vi "CRYMake Calibration Step Default.vi"(8 "Write?":bool, 11 "Hardware flattened":string) -> (3 "Calibration flattened":string)   [LabVIEW 2013]
uses:
  Typedef Control/CRYCalibration 2DCluster.ctl
  Typedef Control/CRYCalibration Cluster.ctl
  Typedef Control/CRYData Cluster.ctl
  Typedef Control/CRYCalibration All Cluster.ctl
  CRYMainGlobal.vi
panel:
  out "OK?":bool
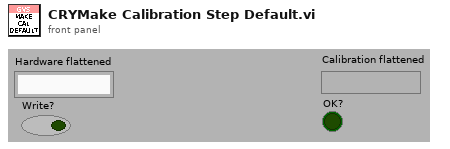
[diagram p1: front panel]
types:
  T1 = typedef "CRYCalibration All Cluster.ctl" = cluster{"Calibration 2D":T2[], "Help":string, "Tab Value":i32, "Input Signal Type":string, "Output Signal Type":string}
  T2 = typedef "CRYCalibration 2DCluster.ctl" = cluster{"Calibration":T3, "Corr Curve":T4, "EQ Curve":T4, "Sens Curve":T4}
  T3 = typedef "CRYCalibration Cluster.ctl" = cluster{"Calibration Step Name":string, "Device":string, "Correction Curve Name":string, "Equalization Curve Name":string, "Sensitivity Curve Name":string, "Corr Folder and File":string, "EQ Folder and File":string, "Sens Folder and File":string, "Corr Step size":u16, "EQ Step size":u16, "Input":bool, "Last Cal Date (sec)":timestamp, "Cha Name":string, "Corr Curve Found":bool, "EQ Curve Found":bool, "Sens Curve Found":bool, "Signal Type":string, "Calibrated Device":string, "Hz":u32}
  T4 = typedef "CRYData Cluster.ctl" = cluster{"Name":string, "Curve":cluster{"x":dbl, "y":dbl, "z":dbl}[], "X data":u16, "Y data":u16, "Z data":u16, "X axis":u16, "Y axis":u16, "Z axis":u16, "X unit":string, "Y unit":string, "Z unit":string, "X dB ref":dbl, "Y dB ref":dbl, "Z dB ref":dbl, "single val":bool, "protected":bool, "display X":bool, "display Y":bool, "display Z":bool, "Test Info":string, "Step No.":i32, "Plot Settings":cluster{"Color":u32, "Interpolation":u8, "Point Style":u8, "Line Style":u8, "Point Color":u32, "Line Width":u8, "Bar Plot Style":u8, "Fill To":i16}, "AutoProtect":bool}
  T5 = cluster{"StepName":string, "setup flattened":string}[]
  T6 = cluster{"StepName":string, "setup flattened":string}
  T7 = enum16{"open", "replace", "create", "open or create", "replace or create", "replace or create with confirmation"}
  T8 = enum16{"big-endian, network order", "native, host order", "little-endian"}
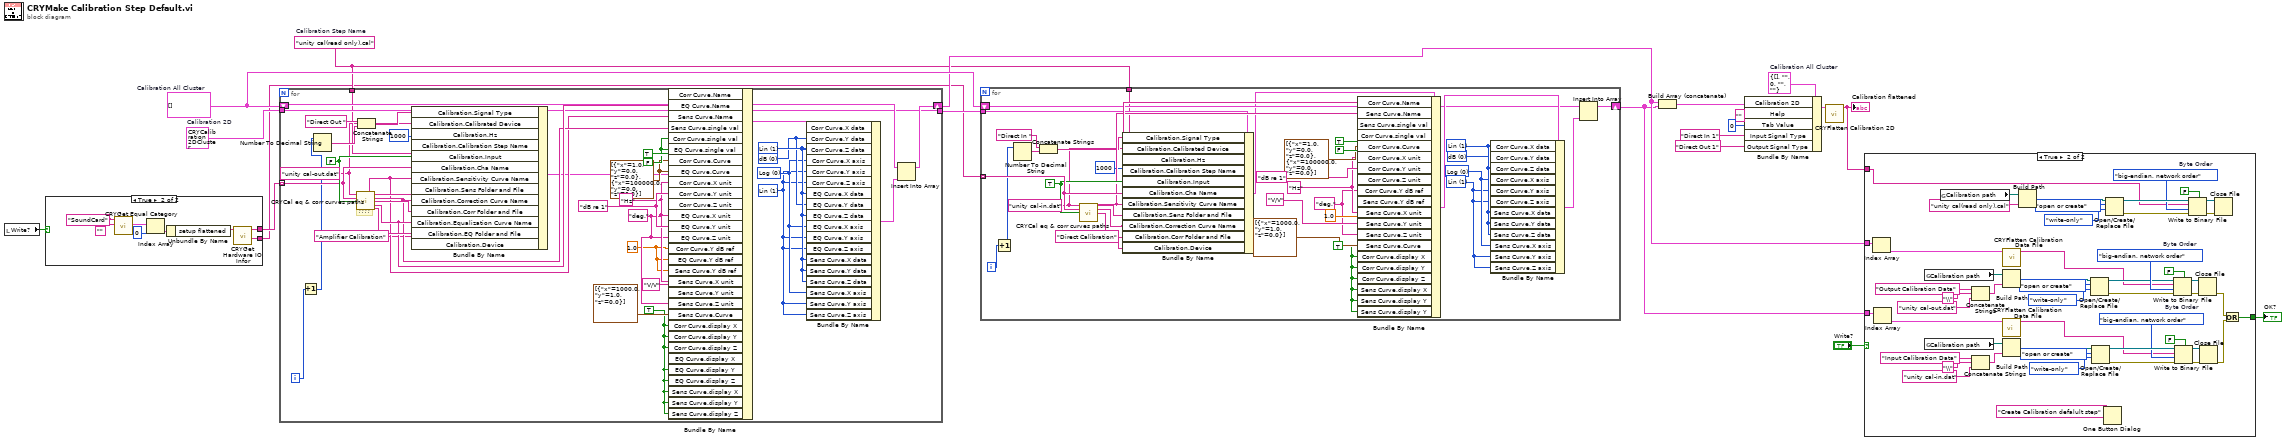
[diagram p0: block diagram]
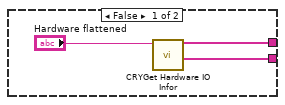
[diagram p2: hidden frame]
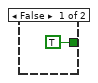
[diagram p3: hidden frame]
diagram:
  w5 = "unity cal(read only).cal"  # Calibration Step Name
  w17 = T1 {"Calibration 2D"=[], "Help"="", "Tab Value"=0, "Input Signal Type"="", "Output Signal Type"=""}  # Calibration All Cluster
  w18 = T2 {"Calibration"={"Calibration Step Name"="", "Device"="", "Correction Curve Name"="", "Equalization Curve Name"="", "Sensitivity Curve Name"="", "Corr Folder and File"="", "EQ Folder and File"="", "Sens Folder and File"="", "Corr Step size"=0, "EQ Step size"=0, "Input"=FALSE, "Last Cal Date (sec)"=timestamp(0 s since 1904-01-01), "Cha Name"="", "Corr Curve Found"=FALSE, "EQ Curve Found"=FALSE, "Sens Curve Found"=FALSE, "Signal Type"="", "Calibrated Device"="", "Hz"=0}, "Corr Curve"={"Name"="", "Curve"=[], "X data"=1, "Y data"=1, "Z data"=1, "X axis"=0, "Y axis"=1, "Z axis"=1, "X unit"="", "Y unit"="", "Z unit"="deg.", "X dB ref"=1.0, "Y dB ref"=1.0, "Z dB ref"=1.0, "single val"=FALSE, "protected"=FALSE, "display X"=FALSE, "display Y"=TRUE, "display Z"=TRUE, "Test Info"="", "Step No."=0, "Plot Settings"={"Color"=0, "Interpolation"=0, "Point Style"=0, "Line Style"=0, "Point Color"=0, "Line Width"=0, "Bar Plot Style"=0, "Fill To"=0}, "AutoProtect"=FALSE}, "EQ Curve"={"Name"="", "Curve"=[], "X data"=1, "Y data"=1, "Z data"=1, "X axis"=0, "Y axis"=1, "Z axis"=1, "X unit"="Hz", "Y unit"="", "Z unit"="deg.", "X dB ref"=1.0, "Y dB ref"=1.0, "Z dB ref"=1.0, "single val"=FALSE, "protected"=FALSE, "display X"=TRUE, "display Y"=TRUE, "display Z"=TRUE, "Test Info"="", "Step No."=0, "Plot Settings"={"Color"=0, "Interpolation"=0, "Point Style"=0, "Line Style"=0, "Point Color"=0, "Line Width"=0, "Bar Plot Style"=0, "Fill To"=0}, "AutoProtect"=FALSE}, "Sens Curve"={"Name"="", "Curve"=[], "X data"=1, "Y data"=1, "Z data"=1, "X axis"=0, "Y axis"=1, "Z axis"=1, "X unit"="Hz", "Y unit"="", "Z unit"="deg.", "X dB ref"=1.0, "Y dB ref"=1.0, "Z dB ref"=1.0, "single val"=FALSE, "protected"=FALSE, "display X"=TRUE, "display Y"=TRUE, "display Z"=TRUE, "Test Info"="", "Step No."=0, "Plot Settings"={"Color"=0, "Interpolation"=0, "Point Style"=0, "Line Style"=0, "Point Color"=0, "Line Width"=0, "Bar Plot Style"=0, "Fill To"=0}, "AutoProtect"=FALSE}}  # Calibration 2D
  w9 = T2[] []  # Calibration All Cluster
  n1 = local read "Write?"() -> (w3:bool)
  n2 = case shown="True" w3 {
    tunnel: [w21 w25] -> w2
    tunnel: [w20 w24] -> w1
    frame False {
      n3 = call "CRYGet Hardware IO Infor.vi"("Hardware setup In"="Hardware flattened") -> ("I_Hardware Channel Name Out"=w20:string[], "O_Hardware Channel Name Out"=w21:string[])  [unwired: 9 out]
    }
    frame True {
      (unwired) ""
      w23 = "SoundCard" ("CategoryName")
      n4 = call "CRYGet Equal Category.vi"("Current StepName"=w23, "Find CategoryName"=w23) -> ("setup flattened Array out"=w27:T5)  [unwired: 9 out]
      n5 = Index Array(array=w27, index=0) -> (element=w28:T6)
      n6 = Unbundle By Name(w28) -> ("setup flattened"=w29:string)
      n7 = call "CRYGet Hardware IO Infor.vi"("Hardware setup In"=w29) -> ("I_Hardware Channel Name Out"=w24:string[], "O_Hardware Channel Name Out"=w25:string[])  [unwired: 9 out]
    }
  }
  n8 = for {
    tunnel: w2 -> [w35] mode=indexing
    shift-right: [w40] -> w7
    shift-left: w9 -> [w41]
    tunnel: w18 -> [w39]
    tunnel: [w39] -> w19
    tunnel: w5 -> [w31]
    i -> [w34]
    w30 = "unity cal-out.dat" ("Step Name")
    w46 = u16 1 items=["Log", "Lin"] ("Y axis")
    w47 = u16 0 items=["Log", "Lin"] ("Y axis")
    w48 = u16 0 items=["dB", "Lin"] ("Y data")
    w49 = u16 1 items=["dB", "Lin"] ("Y data")
    w50 = TRUE ("Corr Curve.display X")
    w56 = 1.0 ("EQ Curve.Y dB ref")
    w57 = "deg." ("Corr Curve.Z unit")
    w60 = "dB re 1" ("Corr Curve.Y unit")
    w59 = "Hz" ("Corr Curve.X unit")
    w61 = cluster{"x":dbl, "y":dbl, "z":dbl}[] [{"x"=1.0, "y"=0.0, "z"=0.0}, {"x"=100000.0, "y"=0.0, "z"=0.0}] ("Corr Curve.Curve")
    w62 = FALSE ("Corr Curve.single val")
    w66 = FALSE ("Input")
    # "????"
    n9 = Increment(x=w34) -> (x+1=w32:i32)
    n10 = Number To Decimal String(number=w32) -> (decimal integer string=w33:string)  [unwired: 1 in]
    n11 = call "CRYCal eq & corr curves paths.vi"("Calibrated Device Name"=w30, "Channel Name"=w35, "In_Out"=w66) -> ("Sens Currve Name"=w51:string, "Sens Curve File"=w65:string, "Corr Curve Name"=w52:string, "Corr Curve File"=w54:string, "EQ Curve Name"=w53:string, "EQ Curve File"=w64:string)  [unwired: 7 out]
    n12 = Concatenate Strings("Direct Out " ("Calibration.Signal Type"), w33) -> (w36:string)
    n13 = Bundle By Name(cluster=w39, "Calibration.Signal Type"=w36, "Calibration.Calibrated Device"=w30, "Calibration.Hz"=u32 1000, "Calibration.Calibration Step Name"=w31, "Calibration.Input"=w66, "Calibration.Cha Name"=w35, "Calibration.Sensitivity Curve Name"=w51, "Calibration.Sens Folder and File"=w65, "Calibration.Correction Curve Name"=w52, "Calibration.Corr Folder and File"=w54, "Calibration.Equalization Curve Name"=w53, "Calibration.EQ Folder and File"=w64, "Calibration.Device"="Amplifier Calibration" ("Device")) -> (w44:T2)
    n14 = Bundle By Name(cluster=w44, "Corr Curve.Name"=w52, "EQ Curve.Name"=w53, "Sens Curve.Name"=w51, "Sens Curve.single val"=TRUE, "Corr Curve.single val"=w62, "EQ Curve.single val"=w62, "Corr Curve.Curve"=w61, "EQ Curve.Curve"=w61, "Corr Curve.X unit"=w59, "Corr Curve.Y unit"=w60, "Corr Curve.Z unit"=w57, "EQ Curve.X unit"=w59, "EQ Curve.Y unit"=w60, "EQ Curve.Z unit"=w57, "Corr Curve.Y dB ref"=w56, "EQ Curve.Y dB ref"=w56, "Sens Curve.Y dB ref"=w56, "Sens Curve.X unit"=w59, "Sens Curve.Y unit"="V/V", "Sens Curve.Z unit"=w57, "Sens Curve.Curve"=cluster{"x":dbl, "y":dbl, "z":dbl}[] [{"x"=1000.0, "y"=1.0, "z"=0.0}], "Corr Curve.display X"=w50, "Corr Curve.display Y"=w50, "Corr Curve.display Z"=w50, "EQ Curve.display X"=w50, "EQ Curve.display Y"=w50, "EQ Curve.display Z"=w50, "Sens Curve.display X"=w50, "Sens Curve.display Y"=w50, "Sens Curve.display Z"=w50) -> (w43:T2)
    n15 = Bundle By Name(cluster=w43, "Corr Curve.X data"=w49, "Corr Curve.Y data"=w48, "Corr Curve.Z data"=w49, "Corr Curve.X axis"=w47, "Corr Curve.Y axis"=w46, "Corr Curve.Z axis"=w46, "EQ Curve.X data"=w49, "EQ Curve.Y data"=w48, "EQ Curve.Z data"=w49, "EQ Curve.X axis"=w47, "EQ Curve.Y axis"=w46, "EQ Curve.Z axis"=w46, "Sens Curve.X data"=w49, "Sens Curve.Y data"=w49, "Sens Curve.Z data"=w49, "Sens Curve.X axis"=w47, "Sens Curve.Y axis"=w46, "Sens Curve.Z axis"=w46) -> (w42:T2)
    n16 = Insert Into Array(array=w41, new element=w42) -> (w40:T2[])  [unwired: 1 in]
  }
  n17 = for {
    tunnel: w1 -> [w101] mode=indexing
    tunnel: w19 -> [w79]
    shift-right: [w77] -> w6
    shift-left: w9 -> [w78]
    tunnel: w5 -> [w69]
    i -> [w75]
    w68 = "unity cal-in.dat" ("Step Name")
    w81 = u16 1 items=["Log", "Lin"] ("Y axis")
    w82 = u16 0 items=["Log", "Lin"] ("Y axis")
    w83 = u16 0 items=["dB", "Lin"] ("Y data")
    w84 = u16 1 items=["dB", "Lin"] ("Y data")
    w86 = TRUE ("Corr Curve.display X")
    w93 = 1.0 ("EQ Curve.Y dB ref")
    w90 = "deg." ("Corr Curve.Z unit")
    w92 = "Hz" ("Corr Curve.X unit")
    w100 = TRUE ("Input")
    n18 = Increment(x=w75) -> (x+1=w70:i32)
    n19 = Number To Decimal String(number=w70) -> (decimal integer string=w74:string)  [unwired: 1 in]
    n20 = Concatenate Strings("Direct In " ("string"), w74) -> (w71:string)
    n21 = call "CRYCal eq & corr curves paths.vi"("Calibrated Device Name"=w68, "Channel Name"=w101, "In_Out"=w100) -> ("Sens Currve Name"=w87:string, "Sens Curve File"=w99:string, "Corr Curve Name"=w88:string, "Corr Curve File"=w98:string)  [unwired: 9 out]
    n22 = Bundle By Name(cluster=w79, "Calibration.Signal Type"=w71, "Calibration.Calibrated Device"=w68, "Calibration.Hz"=u32 1000, "Calibration.Calibration Step Name"=w69, "Calibration.Input"=w100, "Calibration.Cha Name"=w101, "Calibration.Sensitivity Curve Name"=w87, "Calibration.Sens Folder and File"=w99, "Calibration.Correction Curve Name"=w88, "Calibration.Corr Folder and File"=w98, "Calibration.Device"="Direct Calibration" ("Device")) -> (w67:T2)
    n23 = Bundle By Name(cluster=w67, "Corr Curve.Name"=w88, "Sens Curve.Name"=w87, "Sens Curve.single val"=TRUE, "Corr Curve.single val"=FALSE, "Corr Curve.Curve"=cluster{"x":dbl, "y":dbl, "z":dbl}[] [{"x"=1.0, "y"=0.0, "z"=0.0}, {"x"=100000.0, "y"=0.0, "z"=0.0}], "Corr Curve.X unit"=w92, "Corr Curve.Y unit"="dB re 1", "Corr Curve.Z unit"=w90, "Corr Curve.Y dB ref"=w93, "Sens Curve.Y dB ref"=w93, "Sens Curve.X unit"=w92, "Sens Curve.Y unit"="V/V", "Sens Curve.Z unit"=w90, "Sens Curve.Curve"=cluster{"x":dbl, "y":dbl, "z":dbl}[] [{"x"=1000.0, "y"=1.0, "z"=0.0}], "Corr Curve.display X"=w86, "Corr Curve.display Y"=w86, "Corr Curve.display Z"=w86, "Sens Curve.display X"=w86, "Sens Curve.display Y"=w86, "Sens Curve.display Y"=w86) -> (w85:T2)
    n24 = Bundle By Name(cluster=w85, "Corr Curve.X data"=w84, "Corr Curve.Y data"=w83, "Corr Curve.Z data"=w84, "Corr Curve.X axis"=w82, "Corr Curve.Y axis"=w81, "Corr Curve.Z axis"=w81, "Sens Curve.X data"=w84, "Sens Curve.Y data"=w84, "Sens Curve.Z data"=w84, "Sens Curve.X axis"=w82, "Sens Curve.Y axis"=w81, "Sens Curve.Z axis"=w81) -> (w76:T2)
    n25 = Insert Into Array(array=w78, new element=w76) -> (w77:T2[])  [unwired: 1 in]
  }
  n26 = Build Array (concatenate)(w7, w6) -> (w8:T2[])
  n27 = Bundle By Name(cluster=w17, "Calibration 2D"=w8, "Help"="", "Tab Value"=0, "Input Signal Type"="Direct In 1", "Output Signal Type"="Direct Out 1") -> (w16:T1)
  n28 = call "CRYFlatten Calibration 2D.vi"("Calibration All Cluster"=w16) -> ("Calibration flattened"=w4:string)  [unwired: 1 in, 9 out]
  "Calibration flattened" <- w4
  n29 = case shown="True" "Write?" {
    tunnel: w7 -> [_ w152]
    tunnel: w6 -> [_ w150]
    tunnel: [TRUE w116] -> w10
    tunnel: w4 -> [_ w105]
    frame False {
    }
    frame True {
      w107 = T8."big-endian, network order"  # Byte Order
      w122 = T8."big-endian, network order"  # Byte Order
      w147 = T8."big-endian, network order"  # Byte Order
      n30 = Index Array(array=w152) -> (element=w151:T2)  [unwired: 1 in]
      n31 = Index Array(array=w150) -> (element=w149:T2)  [unwired: 1 in]
      n32 = global read "CRYMainGlobal.vi" "Calibration path"() -> (w139:path)
      n33 = global read "CRYMainGlobal.vi" "Calibration path"() -> (w130:path)
      n34 = global read "CRYMainGlobal.vi" "Calibration path"() -> (w114:path)
      n35 = Concatenate Strings("Output Calibration Data" ("string"), "\\" ("string"), "unity cal-out.dat" ("Step File Name")) -> (w140:string)
      n36 = Concatenate Strings("Input Calibration Data" ("string"), "\\" ("string"), "unity cal-in.dat" ("Step File Name")) -> (w129:string)
      n37 = call "CRYFlatten Calibration Data File.vi"("Calibration 2D Cluster"=w149) -> ("Calibration2D flattened"=w120:string)  [unwired: 10 in]
      n38 = call "CRYFlatten Calibration Data File.vi"("Calibration 2D Cluster"=w151) -> ("Calibration2D flattened"=w119:string)  [unwired: 10 in]
      n39 = Build Path(base path=w139, name or relative path=w140) -> (appended path=w138:path)
      n40 = Build Path(base path=w130, name or relative path=w129) -> (appended path=w131:path)
      n41 = Build Path(base path=w114, name or relative path="unity cal(read only).cal" ("string")) -> (appended path=w115:path)
      n42 = Open/Create/Replace File(file path (use dialog)=w138, operation (0:open)=T7."open or create", access (0:read/write)=enum16{"read/write", "read-only", "write-only"}."write-only") -> (refnum out=w144:refnum<file>, error out=w142:errorcluster)  [unwired: 1 in, 3 out]
      n43 = Open/Create/Replace File(file path (use dialog)=w131, operation (0:open)=T7."open or create", access (0:read/write)=enum16{"read/write", "read-only", "write-only"}."write-only") -> (refnum out=w125:refnum<file>, error out=w127:errorcluster)  [unwired: 1 in, 3 out]
      n44 = One Button Dialog(message="Create Calibration defalult step") -> ()  [unwired: 2 out]
      n45 = Open/Create/Replace File(file path (use dialog)=w115, operation (0:open)=T7."open or create", access (0:read/write)=enum16{"read/write", "read-only", "write-only"}."write-only") -> (refnum out=w110:refnum<file>, error out=w112:errorcluster)  [unwired: 1 in, 3 out]
      n46 = Write to Binary File(file (use dialog)=w144, data=w119, error in=w142, 5:FALSE ("prepend array or string size? (T)"), 9:w147) -> (refnum out=w143:refnum<file>, error out=w141:errorcluster)  [unwired: 1 in, 1 out]
      n47 = Write to Binary File(file (use dialog)=w125, data=w120, error in=w127, 5:FALSE ("prepend array or string size? (T)"), 9:w122) -> (refnum out=w126:refnum<file>, error out=w128:errorcluster)  [unwired: 1 in, 1 out]
      n48 = Write to Binary File(file (use dialog)=w110, data=w105, error in=w112, 5:FALSE ("prepend array or string size? (T)"), 9:w107) -> (refnum out=w111:refnum<file>, error out=w113:errorcluster)  [unwired: 1 in, 1 out]
      n49 = Close File(refnum=w143, error in=w141) -> (error out=w118:errorcluster)  [unwired: 1 out]
      n50 = Close File(refnum=w126, error in=w128) -> (error out=w117:errorcluster)  [unwired: 1 out]
      n51 = Close File(refnum=w111, error in=w113) -> ()  [unwired: 2 out]
      n52 = Or(x=w118, y=w117) -> (x .or. y?=w116:bool)
    }
  }
  "OK?" <- w10
